vi "write Cell String to excel location.vi"(8 "error in (no error)":errorcluster, 9 "input string":string, 10 "cell's name":string, 11 "NI_report in":refnum<class "NI_report.lvclass">) -> (0 "error out":errorcluster, 3 "NI_report out":refnum<class "NI_report.lvclass">)   [LabVIEW 2016]
uses:
  <vilib>/Utility/NIReport.llb/NI_report.lvclass
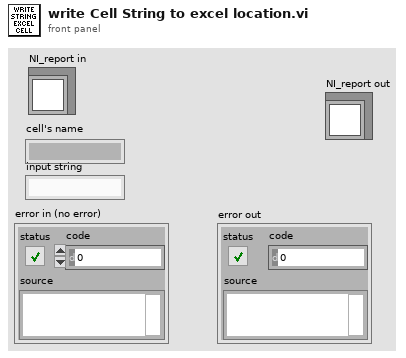
[diagram p1: front panel]
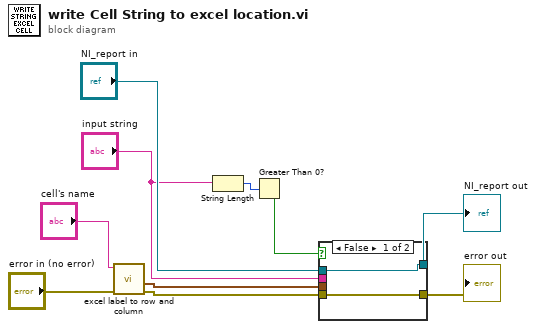
[diagram p0: block diagram]
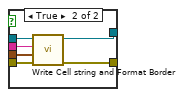
[diagram p2: hidden frame]
diagram:
  n1 = call "excel label to row and column.vi"("error in (no error)"="error in (no error)", "cell's name"="cell's name") -> ("error IO"=w10:errorcluster, "output cluster"=w9:cluster{"row":i32, "column":i32})  [unwired: 5 in, 3 out]
  n2 = String Length(string="input string") -> (length=w2:i32)
  n3 = Greater Than 0?(x=w2) -> (x > 0?=w1:bool)
  n4 = case shown="False" w1 {
    tunnel: w10 -> [w11 w18]
    tunnel: w9 -> [_ w17]
    tunnel: "NI_report in" -> [w12 w16]
    tunnel: [w11 w15] -> w7
    tunnel: [w12 w14] -> w4
    tunnel: "input string" -> [_ w13]
    frame False {
    }
    frame True {
      n5 = call "Write Cell string and Format Border.vi"("error in (no error)"=w18, "output cluster"=w17, "input string"=w13, "NI_report in"=w16) -> ("error out"=w15:errorcluster, "NI_report out"=w14:refnum<class "NI_report.lvclass">)  [unwired: 6 in]
    }
  }
  "error out" <- w7
  "NI_report out" <- w4
